vi "Wattmeter.vi"() -> ()   [LabVIEW 2014]
doc: "This example demonstrates how to continuously acquire buffered voltage measurements using a DAQmx device.\n\nFor instructions on how to connect your signals to the DAQ device, refer to your device documentation."
uses:
  Control 4.ctl
  Control 5.ctl
  <vilib>/Utility/error.llb/DialogType.ctl
  <vilib>/DAQmx/create/channels.llb/DAQmx Create Channel (AI-Voltage-Basic).vi
  <vilib>/DAQmx/configure/timing.llb/DAQmx Timing (Sample Clock).vi
  <vilib>/DAQmx/configure/task.llb/DAQmx Configure Logging (TDMS).vi
  <vilib>/DAQmx/configure/trigger.llb/DAQmx Start Trigger (Digital Edge).vi
  <vilib>/DAQmx/configure/trigger.llb/DAQmx Start Trigger (Analog Edge).vi
  <vilib>/DAQmx/read.llb/DAQmx Read (Analog 1D DBL 1Chan NSamp).vi
  <vilib>/DAQmx/read.llb/DAQmx Read (Analog 1D Wfm NChan NSamp).vi
  <resource>/objmgr/daqmx.rc
panel:
  out "Average Voltage":T1 format="%#_5f"
  in  "DAQmx Physical Channel":tag="Dev2/ai0"
  in  "Stop":bool
  in  "Trigger Type":T2(tab)
  in  "Edge":i32(ring)=10280 items=["Rising"=10280, "Falling"=10171]
  in  "Digital Trigger Source":tag
  in  "Level (V)":dbl format="%0.2f"
  in  "Hysteresis (V)":dbl
  in  "Slope":i32(ring)=10280 items=["Rising"=10280, "Falling"=10171]
  in  "Analog Trigger Source":string="APFI0"
  out "Waveform Graph":waveform(dbl)[](graph)
  in  "TDMS File Path":path
  in  "Number of Samples":i32=100
  in  "Sample Rate":dbl=1000.0
  in  "Sample Clock Source":tag="OnboardClock"
  in  "Terminal Configuration":i32(ring)=10083 items=["default"=-1, "RSE"=10083, "NRSE"=10078, "Differential"=10106, "Pseudodifferential"=12529]
  in  "Max Voltage":dbl=5.0
  in  "Min Voltage":dbl=-5.0
  out "Actual Sample Rate":T3=1000.0 format="%0.2f"
  in  "Logging Mode":i32(ring)=10231 items=["Off"=10231, "Log and Read"=15842]
  # "Channel Settings"
  # "Acquired Data"
  # "Timing Settings"
  # "Trigger Settings"
  # "Logging Settings"
  # "To configure and use a start trigger you must have the necessary tab selected above.  Not all hardware supports triggering--refer to your device documentation for more info."
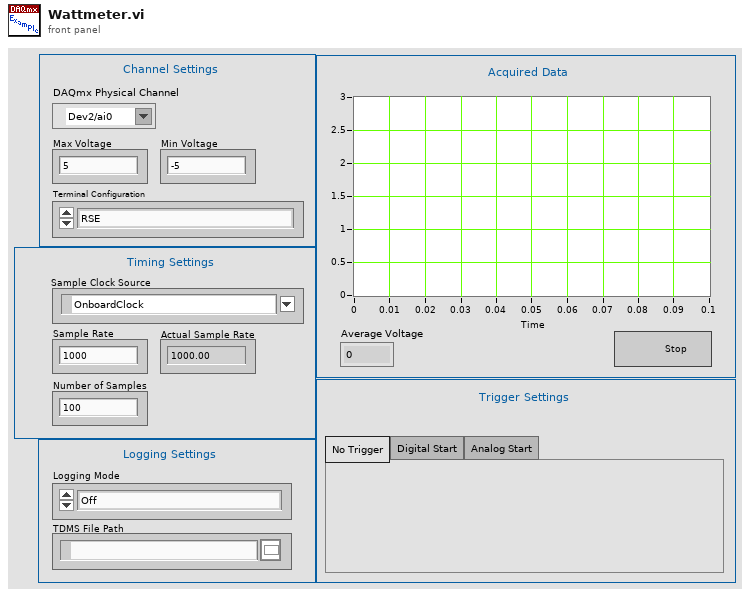
[diagram p1: front panel]
types:
  T1 = typedef "Control 5.ctl" = dbl
  T2 = enum32{"No Trigger", "Digital Start", "Analog Start"}
  T3 = typedef "Control 4.ctl" = dbl
  T4 = typedef "DialogType.ctl" = u16
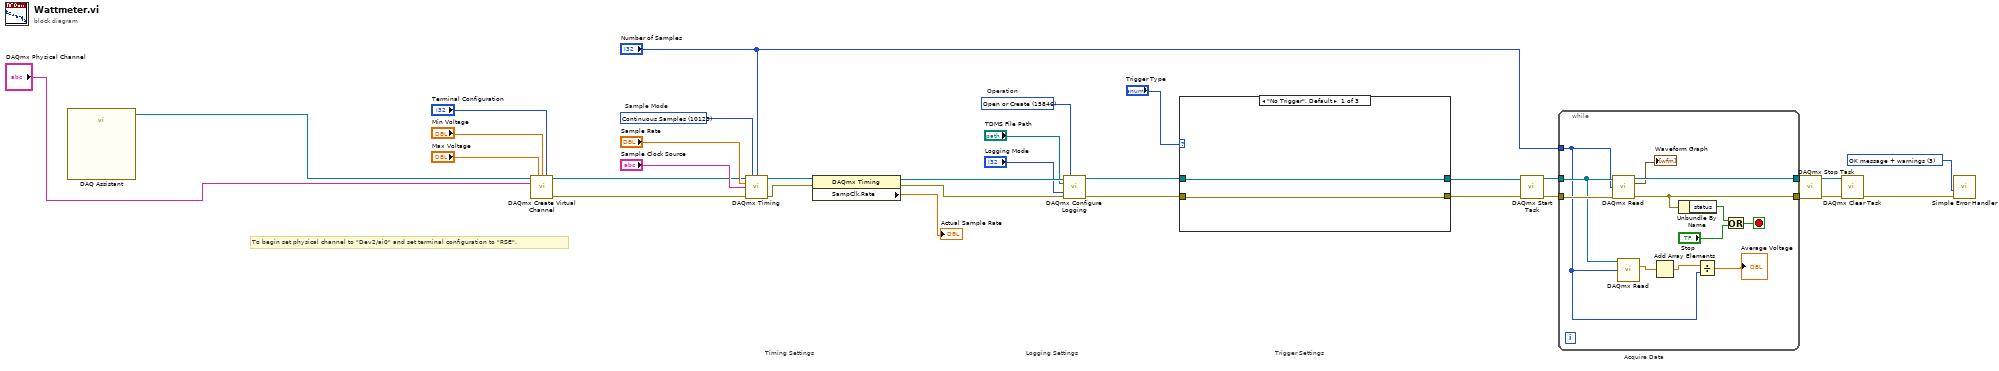
[diagram p0: block diagram]
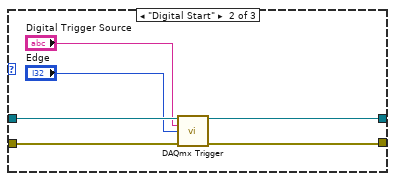
[diagram p2: hidden frame]
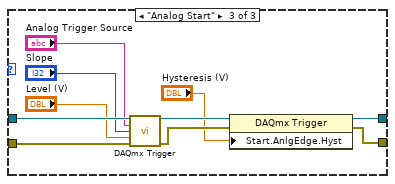
[diagram p3: hidden frame]
diagram:
  w8 = T4 3 items=["no dialog", "OK message", "continue or stop message", "OK message + warnings", "continue/stop + warnings"] ("type of dialog (OK msg:1)")
  w27 = 15846 items=["Open"=10437, "Open or Create"=15846, "Create or Replace"=15847, "Create"=15848]  # Operation
  w30 = 10123 items=["Finite Samples"=10178, "Continuous Samples"=10123, "Hardware Timed Single Point"=12522]  # Sample Mode
  # "To begin set physical channel to \"Dev2/ai0\" and set terminal configuration to \"RSE\"."
  # "Acquire Data"
  # "Trigger Settings"
  # "Timing Settings"
  # "Logging Settings"
  n1 = call "DAQ Assistant"() -> ("task out"=w2:refnum<k21>)  [unwired: 17 in, 2 out]
  n2 = call-poly <vilib>:"DAQmx Create Virtual Channel.vi"("task in"=w2, "maximum value"="Max Voltage", "minimum value"="Min Voltage", "input terminal configuration"="Terminal Configuration", "physical channels"="DAQmx Physical Channel") -> ("task out"=w3:refnum<k21>, "error out"=w4:errorcluster)  [unwired: 9 in]
  n3 = call-poly <vilib>:"DAQmx Timing.vi"("task/channels in"=w3, "sample mode"=w30, "samples per channel"="Number of Samples", "rate"="Sample Rate", "source"="Sample Clock Source", "error in"=w4) -> ("task out"=w32:refnum<k21>, "error out"=w31:errorcluster)  [unwired: 8 in]
  n4 = property class="DAQmx Timing"(reference=w32, error in=w31) -> (reference out=w29:refnum<k21>, error out=w28:errorcluster, "SampClk.Rate"=→"Actual Sample Rate":dbl)
  n5 = call-poly <vilib>:"DAQmx Configure Logging.vi"("task/channels in"=w29, "operation"=w27, "file path"="TDMS File Path", "logging mode"="Logging Mode", "error in"=w28) -> ("task out"=w26:refnum<k21>, "error out"=w25:errorcluster)  [unwired: 9 in]
  n6 = case shown="\"No Trigger\", Default" "Trigger Type" {
    tunnel: w26 -> [w34 w40 w50]
    tunnel: w25 -> [w33 w39 w49]
    tunnel: [w34 w38 w47] -> w24
    tunnel: [w33 w37 w46] -> w23
    frame "No Trigger", Default {
    }
    frame "Digital Start" {
      n7 = call-poly <vilib>:"DAQmx Trigger.vi"("task/channels in"=w40, "source"="Digital Trigger Source", "edge"="Edge", "error in"=w39) -> ("task out"=w38:refnum<k21>, "error out"=w37:errorcluster)  [unwired: 10 in]
    }
    frame "Analog Start" {
      n8 = call-poly <vilib>:"DAQmx Trigger.vi"("task/channels in"=w50, "source"="Analog Trigger Source", "slope"="Slope", "level"="Level (V)", "error in"=w49) -> ("task out"=w45:refnum<k21>, "error out"=w44:errorcluster)  [unwired: 9 in]
      n9 = property class="DAQmx Trigger"(reference=w45, error in=w44, "Start.AnlgEdge.Hyst"="Hysteresis (V)") -> (reference out=w47:refnum<k21>, error out=w46:errorcluster)
    }
  }
  n10 = call <vilib>:"DAQmx Start Task.vi"("task/channels in"=w24, "error in"=w23) -> ("task out"=w22:refnum<k21>, "error out"=w21:errorcluster)  [unwired: 12 in]
  n11 = while {
    tunnel: w22 -> [w55]
    tunnel: w21 -> [w57]
    tunnel: [w62] -> w12
    tunnel: [w60] -> w11
    tunnel: "Number of Samples" -> [w52]
    stop <- w58 stop-if-true
    n12 = call-poly <vilib>:"DAQmx Read.vi"("task/channels in"=w55, "number of samples per channel"=w52, "error in"=w57) -> ("task out"=w62:refnum<k21>, "data"=→"Waveform Graph":waveform(dbl)[], "error out"=w60:errorcluster)  [unwired: 10 in]
    n13 = call-poly <vilib>:"DAQmx Read.vi"("task/channels in"=w55, "number of samples per channel"=w52) -> ("data"=w54:dbl[])  [unwired: 11 in, 2 out]
    n14 = Add Array Elements(numeric array=w54) -> (sum=w53:dbl)
    n15 = Unbundle By Name(w60) -> ("status"=w59:bool)
    n16 = Divide(x=w53, y=w52) -> (x/y=→"Average Voltage":dbl)
    n17 = Or(x=w59, y="Stop") -> (x .or. y?=w58:bool)
  }
  n18 = call <vilib>:"DAQmx Stop Task.vi"("task/channels in"=w12, "error in"=w11) -> ("task out"=w9:refnum<k21>, "error out"=w10:errorcluster)  [unwired: 12 in]
  n19 = call <vilib>:"DAQmx Clear Task.vi"("task in"=w9, "error in"=w10) -> ("error out"=w20:errorcluster)  [unwired: 13 in]
  n20 = call <vilib>:"Simple Error Handler.vi"("type of dialog (OK msg:1)"=w8, "error in (no error)"=w20) -> ()  [unwired: 3 in, 5 out]
